vi "input.vi"(8 "error in":errorcluster, 10 "data table in":T1, 11 "EthernetIP runtime in":refnum<class "EIP Tags Runtime.lvclass">) -> (0 "error out":errorcluster, 2 "data table out":T1, 3 "EthernetIP runtime out":refnum<class "EIP Tags Runtime.lvclass">)   [LabVIEW 2013, in "EIP Tags Runtime.lvclass"]
doc: "Provides an interface for reading data from a module at runtime. While this interface performs no operations, a child should provide an override which may read from any open sessions, references, or interfaces."
uses:
  EIP Tags Runtime.lvclass
  <vilib>/NI/Tag Bus/table/data table.ctl
  EIP Tags Runtime.lvclass/EIP Tags Runtime.ctl
  <vilib>/NI/Tag Bus/table/data polymorphs/write many/write I8s.vi
  <vilib>/NI/Tag Bus/table/data polymorphs/write many/write I16s.vi
  <vilib>/NI/Tag Bus/table/data polymorphs/write many/write I32s.vi
  <vilib>/NI/Tag Bus/table/data polymorphs/write many/write Singles.vi
  <vilib>/NI/Tag Bus/table/data polymorphs/write many/write Booleans.vi
  <vilib>/NI/Tag Bus/table/data polymorphs/write one/write String.vi
  <vilib>/ethernetip/ethernetip.llb/EthernetIP Tag Read SINT.vi
  <vilib>/ethernetip/ethernetip.llb/EthernetIP Tag Read INT.vi
  <vilib>/ethernetip/ethernetip.llb/EthernetIP Tag Read DINT.vi
  <vilib>/ethernetip/ethernetip.llb/EthernetIP Tag Read REAL.vi
  <vilib>/ethernetip/ethernetip.llb/EthernetIP Tag Read BOOL.vi
  <vilib>/ethernetip/ethernetip.llb/EthernetIP Tag Read STRING.vi
  <vilib>/ethernetip/ethernetip.lvlib
  <vilib>/NI/Tag Bus/table/data table.lvlib
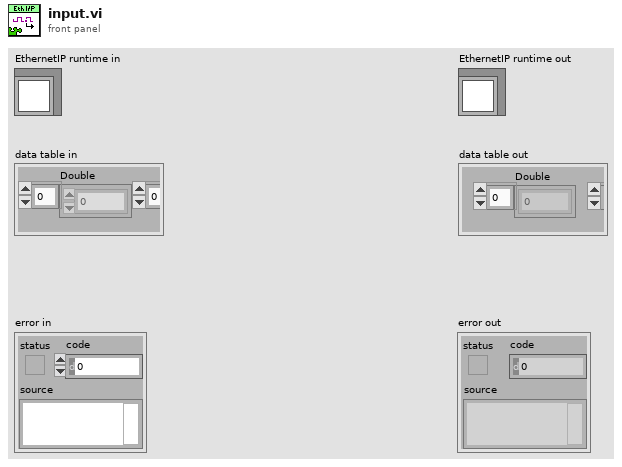
[diagram p1: front panel]
types:
  T1 = typedef "tag bus.lvlib/data table.lvlib/data table.ctl" = cluster{"Double":dbl[], "Single":sgl[], "I64":i64[], "I32":i32[], "I16":i16[], "I8":i8[], "U64":u64[], "U32":u32[], "U16":u16[], "U8":u8[], "Boolean":bool[], "String":string[], "Array of Double":cluster{"DBL Array":dbl[]}[], "Array of Single":cluster{"SGL Array":sgl[]}[], "Array of I64":cluster{"I64 Array":i64[]}[], "Array of I32":cluster{"I32 Array":i32[]}[], "Array of I16":cluster{"I16 Array":i16[]}[], "Array of I8":cluster{"I8 Array":i8[]}[], "Array of U64":cluster{"U64 Array":u64[]}[], "Array of U32":cluster{"U32 Array":u32[]}[], "Array of U16":cluster{"U16 Array":u16[]}[], "Array of U8":cluster{"U8 Array":u8[]}[], "Array of Boolean":cluster{"Boolean Array":bool[]}[], "Array of String":cluster{"String Array":string[]}[]}
  T2 = typedef "ethernetip.lvlib/ethernetip.ctl" = refnum<k21>
  T3 = typedef "EIP Tags Runtime.lvclass/eip tag spec.ctl" = cluster{"eip tag types":T4, "Network Path":string, "Tag Name":string, "Number of Elements":u32, "data indices":i32[], "tag bus indices":i32[]}
  T4 = typedef "EIP Tags Configuration.lvclass/eip tag types.ctl" = enum16{"SINT", "INT", "DINT", "REAL", "BOOL", "STRING"}
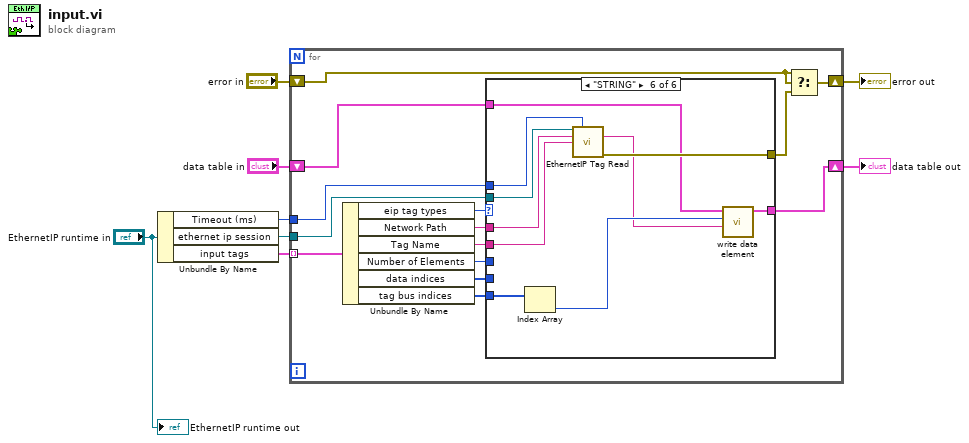
[diagram p0: block diagram]
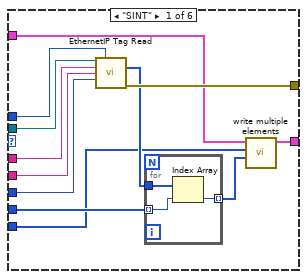
[diagram p2: hidden frame]
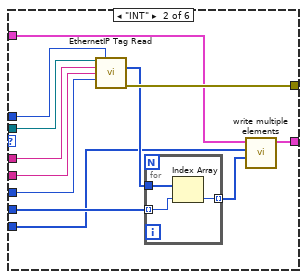
[diagram p3: hidden frame]
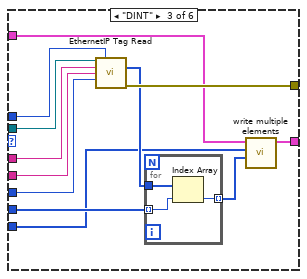
[diagram p4: hidden frame]
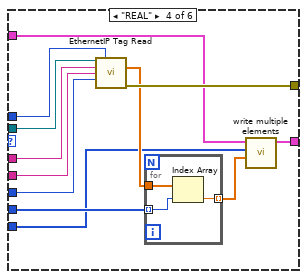
[diagram p5: hidden frame]
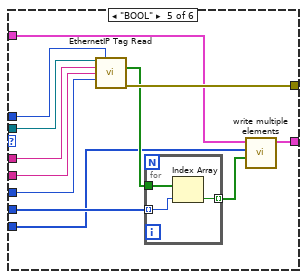
[diagram p6: hidden frame]
diagram:
  n1 = Unbundle By Name("EthernetIP runtime in") -> ("Timeout (ms)"=w1:i32, "ethernet ip session"=w7:T2, "input tags"=w4:T3[])
  n2 = for {
    tunnel: w7 -> [w18]
    shift-right: [w21] -> w5
    shift-left: "error in" -> [w22]
    tunnel: w4 -> [w20] mode=indexing
    shift-right: [w14] -> w2
    shift-left: "data table in" -> [w15]
    tunnel: w1 -> [w17]
    n3 = Unbundle By Name(w20) -> ("eip tag types"=w19:T4, "Network Path"=w13:string, "Tag Name"=w12:string, "Number of Elements"=w11:u32, "data indices"=w10:i32[], "tag bus indices"=w9:i32[])
    n4 = case shown="\"STRING\"" w19 {
      tunnel: w18 -> [w34 w49 w64 w79 w94 w107]
      tunnel: w17 -> [w33 w48 w63 w78 w93 w106]
      tunnel: [w32 w47 w62 w77 w92 w105] -> w16
      tunnel: w15 -> [w25 w40 w55 w70 w85 w101]
      tunnel: [w26 w41 w56 w71 w86 w102] -> w14
      tunnel: w13 -> [w31 w46 w61 w76 w91 w104]
      tunnel: w12 -> [w30 w45 w60 w75 w90 w103]
      tunnel: w11 -> [w29 w44 w59 w74 w89 _]
      tunnel: w10 -> [w27 w42 w57 w72 w87 _]
      tunnel: w9 -> [w23 w38 w53 w68 w83 w100]
      frame "SINT" {
        n5 = call-poly <vilib>:"EthernetIP Tag Read.vi"("Session in"=w34, "Timeout (ms)"=w33, "Network Path"=w31, "Tag Name"=w30, "Number of Elements"=w29) -> ("Data"=w28:i8[], "error out"=w32:errorcluster)  [unwired: 8 in, 1 out]
        n6 = for {
          tunnel: w28 -> [w37]
          tunnel: w27 -> [w36] mode=indexing
          tunnel: [w35] -> w24 mode=indexing
          n7 = Index Array(array=w37, index=w36) -> (element=w35:i8)
        }
        n8 = call-poly <vilib>:"write multiple elements.vi"("values"=w24, "indices"=w23, "data table in"=w25) -> ("data table out"=w26:T1)  [unwired: 8 in]
      }
      frame "INT" {
        n9 = call-poly <vilib>:"EthernetIP Tag Read.vi"("Session in"=w49, "Timeout (ms)"=w48, "Network Path"=w46, "Tag Name"=w45, "Number of Elements"=w44) -> ("Data"=w43:i16[], "error out"=w47:errorcluster)  [unwired: 8 in, 1 out]
        n10 = for {
          tunnel: w43 -> [w52]
          tunnel: w42 -> [w51] mode=indexing
          tunnel: [w50] -> w39 mode=indexing
          n11 = Index Array(array=w52, index=w51) -> (element=w50:i16)
        }
        n12 = call-poly <vilib>:"write multiple elements.vi"("values"=w39, "indices"=w38, "data table in"=w40) -> ("data table out"=w41:T1)  [unwired: 8 in]
      }
      frame "DINT" {
        n13 = call-poly <vilib>:"EthernetIP Tag Read.vi"("Session in"=w64, "Timeout (ms)"=w63, "Network Path"=w61, "Tag Name"=w60, "Number of Elements"=w59) -> ("Data"=w58:i32[], "error out"=w62:errorcluster)  [unwired: 8 in, 1 out]
        n14 = for {
          tunnel: w58 -> [w67]
          tunnel: w57 -> [w66] mode=indexing
          tunnel: [w65] -> w54 mode=indexing
          n15 = Index Array(array=w67, index=w66) -> (element=w65:i32)
        }
        n16 = call-poly <vilib>:"write multiple elements.vi"("values"=w54, "indices"=w53, "data table in"=w55) -> ("data table out"=w56:T1)  [unwired: 8 in]
      }
      frame "REAL" {
        n17 = call-poly <vilib>:"EthernetIP Tag Read.vi"("Session in"=w79, "Timeout (ms)"=w78, "Network Path"=w76, "Tag Name"=w75, "Number of Elements"=w74) -> ("Data"=w73:sgl[], "error out"=w77:errorcluster)  [unwired: 8 in, 1 out]
        n18 = for {
          tunnel: w73 -> [w82]
          tunnel: w72 -> [w81] mode=indexing
          tunnel: [w80] -> w69 mode=indexing
          n19 = Index Array(array=w82, index=w81) -> (element=w80:sgl)
        }
        n20 = call-poly <vilib>:"write multiple elements.vi"("values"=w69, "indices"=w68, "data table in"=w70) -> ("data table out"=w71:T1)  [unwired: 8 in]
      }
      frame "BOOL" {
        n21 = call-poly <vilib>:"EthernetIP Tag Read.vi"("Session in"=w94, "Timeout (ms)"=w93, "Network Path"=w91, "Tag Name"=w90, "Number of Elements"=w89) -> ("Data"=w88:bool[], "error out"=w92:errorcluster)  [unwired: 8 in, 1 out]
        n22 = for {
          tunnel: w88 -> [w97]
          tunnel: w87 -> [w96] mode=indexing
          tunnel: [w95] -> w84 mode=indexing
          n23 = Index Array(array=w97, index=w96) -> (element=w95:bool)
        }
        n24 = call-poly <vilib>:"write multiple elements.vi"("values"=w84, "indices"=w83, "data table in"=w85) -> ("data table out"=w86:T1)  [unwired: 8 in]
      }
      frame "STRING" {
        n25 = Index Array(array=w100) -> (element=w99:i32)  [unwired: 1 in]
        n26 = call-poly <vilib>:"EthernetIP Tag Read.vi"("Session in"=w107, "Timeout (ms)"=w106, "Network Path"=w104, "Tag Name"=w103) -> ("Data"=w98:string, "error out"=w105:errorcluster)  [unwired: 9 in, 1 out]
        n27 = call-poly <vilib>:"write data element.vi"("value"=w98, "index"=w99, "data table in"=w101) -> ("data table out"=w102:T1)  [unwired: 8 in]
      }
    }
    n28 = Select(t=w22, s=w22, f=w16) -> (s? t:f=w21:errorcluster)
  }
  "error out" <- w5
  "data table out" <- w2
  "EthernetIP runtime out" <- "EthernetIP runtime in"
